vi "FL_React_on_incoming_TTLs.vi"(0 "IO parameters in":T3, 5 "Data in":T1, 7 "Notifier in":refnum<notifier>, 9 "Queue in":refnum<queue>, 11 "error in (no error)":T4) -> (3 "TTL received at (HW)":u32, 4 "TTL received at (SW)":timestamp, 6 "Data out":T1, 8 "Notifier out":refnum<notifier>, 10 "Queue out":refnum<queue>, 15 "error out":errorcluster)   [LabVIEW 2018, in "Tracker.lvlib"]
uses:
  Tracker.lvlib
  Controls/CTL_States_cluster.ctl
  Controls/CTL_Control_States.ctl
  Controls/CTL_IO_params_cluster.ctl
  Controls/CTL_Full_data_frame.ctl
  Controls/CTL_Animal_Coordinates_and_Speed.ctl
  <vilib>/ptbypt/NI_PtbyPt.lvlib
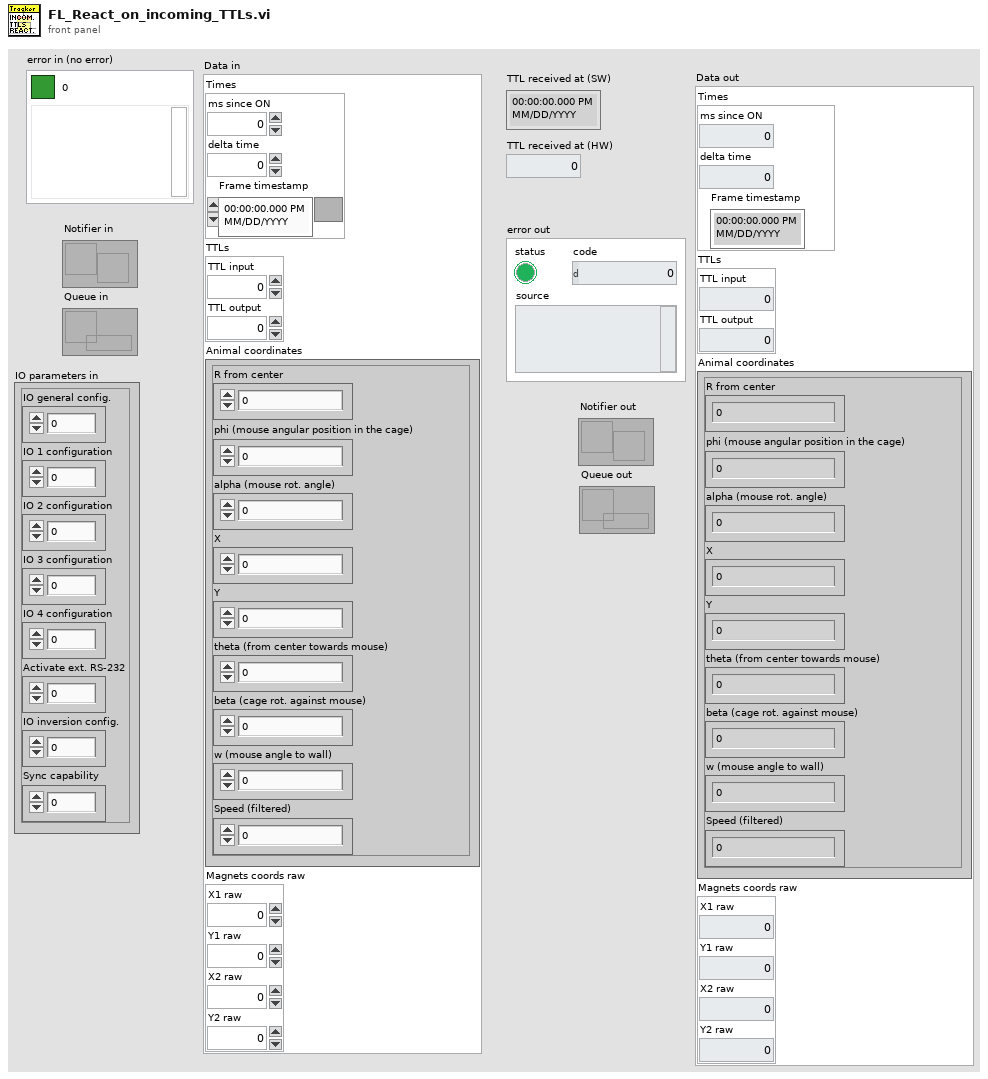
[diagram p1: front panel]
types:
  T1 = typedef "Tracker.lvlib/CTL_Full_data_frame.ctl" = cluster{"Times":cluster{"ms since ON":u32, "delta time":u32, "Frame timestamp":timestamp}, "TTLs":cluster{"TTL input":i16, "TTL output":i16}, "Animal coordinates":T2, "Magnets coords raw":cluster{"X1 raw":dbl, "Y1 raw":dbl, "X2 raw":dbl, "Y2 raw":dbl}}
  T2 = typedef "Tracker.lvlib/CTL_Animal_Coordinates_and_Speed.ctl" = cluster{"R from center":dbl, "phi (mouse angular position in the cage)":dbl, "alpha (mouse rot. angle)":sgl, "X":dbl, "Y":dbl, "theta (from center towards mouse)":dbl, "beta (cage rot. against mouse)":sgl, "w (mouse angle to wall)":dbl, "Speed (filtered)":dbl}
  T3 = typedef "Tracker.lvlib/CTL_IO_params_cluster.ctl" = cluster{"IO general config.":u16, "IO 1 configuration":u16, "IO 2 configuration":u16, "IO 3 configuration":u16, "IO 4 configuration":u16, "Activate ext. RS-232":u16, "IO inversion config.":u16, "Sync capability":u8}
  T4 = cluster{"Boolean Round":bool, "code":i32, "source":string}
  T5 = typedef "Tracker.lvlib/CTL_States_cluster.ctl" = cluster{"Acq. is ON":bool, "Playing loaded":bool, "Recording now":bool, "Has been recorded":bool, "Data saved":bool, "Data loaded":bool, "Calibration mode":bool, "Offline mode":bool, "Stop and Exit":bool}
  T6 = typedef "Tracker.lvlib/CTL_Control_States.ctl" = enum16{"SW Init", "HW Init", "Close App", "Update port info (Init OK)", "Unlock UI (init OK)", "Save HW Settings", "Re-check HW (init failed)", "Configure port(s)", "Switch to Offline mode", "Zones layout update", "Set I/O config", "Reset stimulus", "Reset zones", "Play Start", "Play Stop", "Upd. FPS", "Upd. trace length", "Cage and recording settings", "Update filter", "Timings calibration start", "Timings calibration finish", "Dispension calibration", "Save all settings", "Start Recording", "Stop Recording", "Recording post-processing", "Load recorded data"}
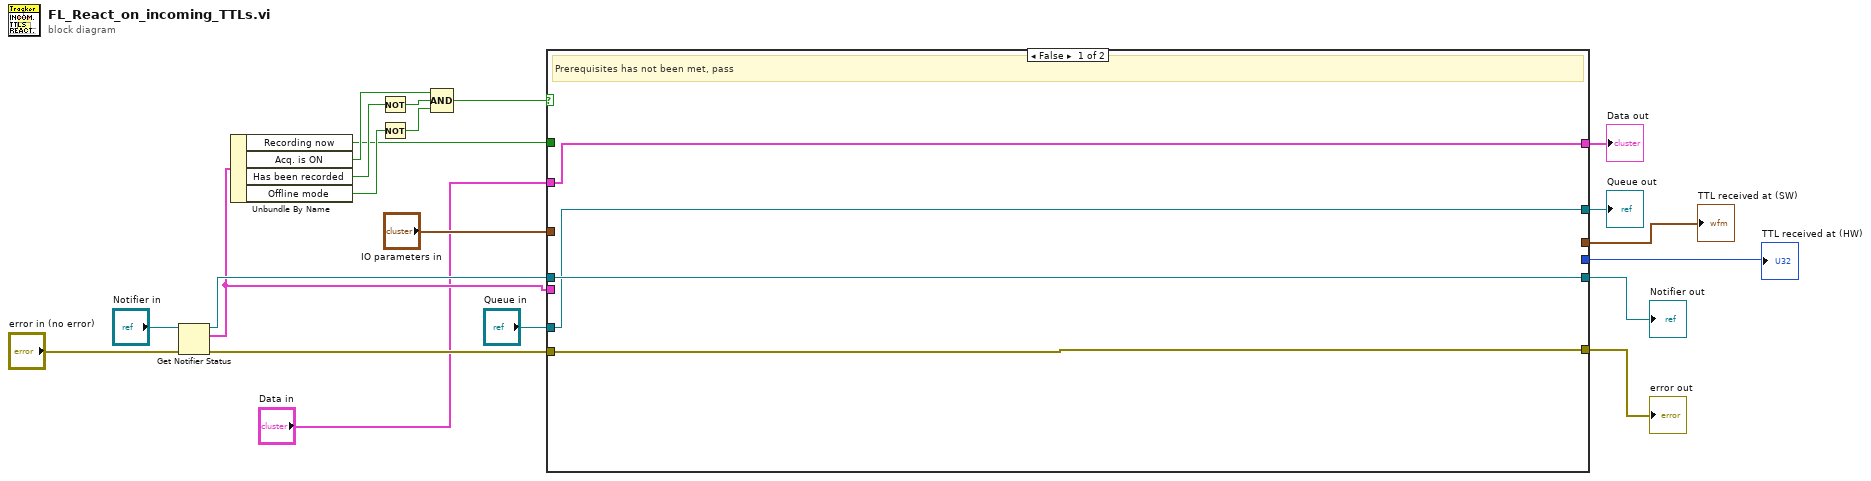
[diagram p0: block diagram]
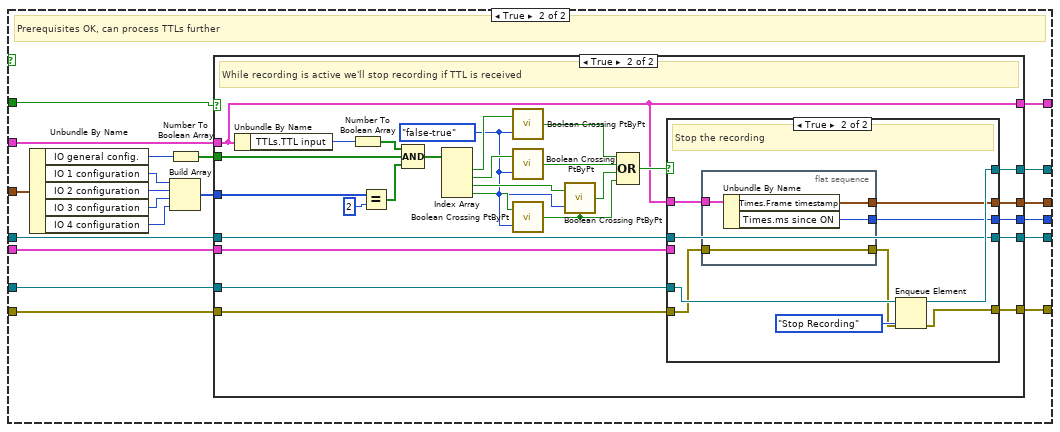
[diagram p2: hidden frame]
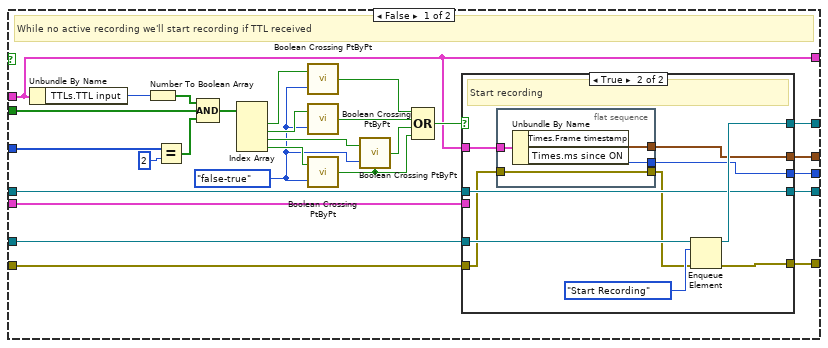
[diagram p3: hidden frame]
diagram:
  n1 = Get Notifier Status(notifier="Notifier in", error in (no error)="error in (no error)") -> (notifier out=w11:refnum<notifier>, current notification=w5:T5, error out=w13:errorcluster)  [unwired: 2 out]
  n2 = Unbundle By Name(w5) -> ("Recording now"=w8:bool, "Acq. is ON"=w19:bool, "Has been recorded"=w17:bool, "Offline mode"=w15:bool)
  n3 = Not(x=w17) -> (.not. x?=w16:bool)
  n4 = Not(x=w15) -> (.not. x?=w14:bool)
  n5 = Compound Arithmetic op=AND(w19, w16, w14) -> (w18:bool)
  n6 = case shown="False" w18 {
    tunnel: w13 -> [w25 w33]
    tunnel: [w25 w31] -> w12
    tunnel: "Data in" -> [w24 w29]
    tunnel: [w24 w28] -> w2
    tunnel: w11 -> [w23 w36]
    tunnel: [w23 w34] -> w6
    tunnel: "Queue in" -> [w22 w32]
    tunnel: [w22 w30] -> w9
    tunnel: w8 -> [_ w45]
    tunnel: "IO parameters in" -> [_ w43]
    tunnel: w5 -> [_ w35]
    tunnel: [_ w27] -> w4
    tunnel: [_ w26] -> w1
    frame False {
      # "Prerequisites has not been met, pass"
    }
    frame True {
      # "Prerequisites OK, can process TTLs further"
      n7 = Unbundle By Name(w43) -> ("IO general config."=w44:u16, "IO 1 configuration"=w42:u16, "IO 2 configuration"=w41:u16, "IO 3 configuration"=w40:u16, "IO 4 configuration"=w39:u16)
      n8 = Build Array(w42, w41, w40, w39) -> (w38:u16[])
      n9 = Number To Boolean Array(number=w44) -> (Boolean array=w37:bool[])
      n10 = case shown="True" w45 {
        tunnel: w38 -> [w71 w96]
        tunnel: w37 -> [w72 w97]
        tunnel: w36 -> [w66 w112]
        tunnel: w35 -> [w65 w111]
        tunnel: [w64 w110] -> w34
        tunnel: w33 -> [w68 w114]
        tunnel: w32 -> [w70 w116]
        tunnel: [w69 w115] -> w31
        tunnel: [w67 w113] -> w30
        tunnel: w29 -> [w47 w91]
        tunnel: [w47 w91] -> w28
        tunnel: [w48 w92] -> w27
        tunnel: [w46 w90] -> w26
        frame False {
          w53 = enum16{"either", "false-true", "true-false"}."false-true" ("direction")
          # "While no active recording we'll start recording if TTL received"
          n11 = Unbundle By Name(w47) -> ("TTLs.TTL input"=w50:i16)
          n12 = Number To Boolean Array(number=w50) -> (Boolean array=w49:bool[])
          n13 = Equal?(x=w71, y=u16 2) -> (x = y?=w62:bool[])
          n14 = Compound Arithmetic op=AND(w49, w72, w62) -> (w61:bool[])
          n15 = Index Array(array=w61) -> (element #1=w60:bool, element #2=w56:bool, element #3=w55:bool, element #4=w54:bool)  [unwired: 4 in]
          n16 = call <vilib>:"Boolean Crossing PtByPt.vi"("direction"=w53, "input"=w60) -> ("crossing"=w58:bool)  [unwired: 1 in]
          n17 = call <vilib>:"Boolean Crossing PtByPt.vi"("direction"=w53, "input"=w56) -> ("crossing"=w57:bool)  [unwired: 1 in]
          n18 = call <vilib>:"Boolean Crossing PtByPt.vi"("direction"=w53, "input"=w54) -> ("crossing"=w51:bool)  [unwired: 1 in]
          n19 = call <vilib>:"Boolean Crossing PtByPt.vi"("initialize"=w51, "direction"=w53, "input"=w55) -> ("crossing"=w52:bool)
          n20 = Compound Arithmetic op=OR(w58, w57, w52, w51) -> (w59:bool)
          n21 = case shown="True" w59 {
            tunnel: w70 -> [w74 w85]
            tunnel: [w75 w81] -> w69
            tunnel: w68 -> [w75 w79]
            tunnel: [w74 w83] -> w67
            tunnel: w66 -> [w73 w82]
            tunnel: w65 -> [_ _]
            tunnel: [w73 w82] -> w64
            tunnel: [_ w80] -> w48
            tunnel: w47 -> [_ w77]
            tunnel: [_ w76] -> w46
            frame False {
            }
            frame True {
              # "Start recording"
              n22 = flat-sequence {
                tunnel: [w87] -> w80
                tunnel: w79 -> [w89]
                tunnel: [w89] -> w78
                tunnel: w77 -> [w88]
                tunnel: [w86] -> w76
                frame #0 {
                  n23 = Unbundle By Name(w88) -> ("Times.Frame timestamp"=w87:timestamp, "Times.ms since ON"=w86:u32)
                }
              }
              n24 = Enqueue Element(queue=w85, element=CTL_Control_States."Start Recording", error in (no error)=w78) -> (queue out=w83:refnum<queue>, error out=w81:errorcluster)  [unwired: 1 in, 1 out]
            }
          }
        }
        frame True {
          w99 = enum16{"either", "false-true", "true-false"}."false-true" ("direction")
          # "While recording is active we'll stop recording if TTL is received"
          n25 = Unbundle By Name(w91) -> ("TTLs.TTL input"=w94:i16)
          n26 = Number To Boolean Array(number=w94) -> (Boolean array=w93:bool[])
          n27 = Equal?(x=w96, y=u16 2) -> (x = y?=w109:bool[])
          n28 = Compound Arithmetic op=AND(w93, w97, w109) -> (w108:bool[])
          n29 = Index Array(array=w108) -> (element #1=w107:bool, element #2=w104:bool, element #3=w103:bool, element #4=w102:bool)  [unwired: 4 in]
          n30 = call <vilib>:"Boolean Crossing PtByPt.vi"("direction"=w99, "input"=w107) -> ("crossing"=w106:bool)  [unwired: 1 in]
          n31 = call <vilib>:"Boolean Crossing PtByPt.vi"("direction"=w99, "input"=w104) -> ("crossing"=w105:bool)  [unwired: 1 in]
          n32 = call <vilib>:"Boolean Crossing PtByPt.vi"("direction"=w99, "input"=w102) -> ("crossing"=w100:bool)  [unwired: 1 in]
          n33 = call <vilib>:"Boolean Crossing PtByPt.vi"("initialize"=w100, "direction"=w99, "input"=w103) -> ("crossing"=w101:bool)
          n34 = Compound Arithmetic op=OR(w106, w105, w101, w100) -> (w95:bool)
          n35 = case shown="True" w95 {
            tunnel: w116 -> [w118 w129]
            tunnel: [w119 w126] -> w115
            tunnel: w114 -> [w119 w123]
            tunnel: [w118 w127] -> w113
            tunnel: w112 -> [w117 w125]
            tunnel: w111 -> [_ _]
            tunnel: [w117 w125] -> w110
            tunnel: [_ w124] -> w92
            tunnel: w91 -> [_ w121]
            tunnel: [_ w120] -> w90
            frame False {
            }
            frame True {
              # "Stop the recording"
              n36 = flat-sequence {
                tunnel: [w131] -> w124
                tunnel: w123 -> [w133]
                tunnel: [w133] -> w122
                tunnel: w121 -> [w132]
                tunnel: [w130] -> w120
                frame #0 {
                  n37 = Unbundle By Name(w132) -> ("Times.Frame timestamp"=w131:timestamp, "Times.ms since ON"=w130:u32)
                }
              }
              n38 = Enqueue Element(queue=w129, element=CTL_Control_States."Stop Recording", error in (no error)=w122) -> (queue out=w127:refnum<queue>, error out=w126:errorcluster)  [unwired: 1 in, 1 out]
            }
          }
        }
      }
    }
  }
  "error out" <- w12
  "Notifier out" <- w6
  "Queue out" <- w9
  "TTL received at (SW)" <- w4
  "Data out" <- w2
  "TTL received at (HW)" <- w1
